vi "FindAltName_wPostfix.vi"(10 "Token":string="__", 11 "File Path Control in":path) -> (3 "File Path Control out":path)   [LabVIEW 2013, in "TestVIs.lvlib"]
doc: "Strips any postfix name from a filename/path. All characters following (and including) the token string are removed. Any file extension is preserved. Token defaults to double-underscore."
uses:
  TestVIs.lvlib
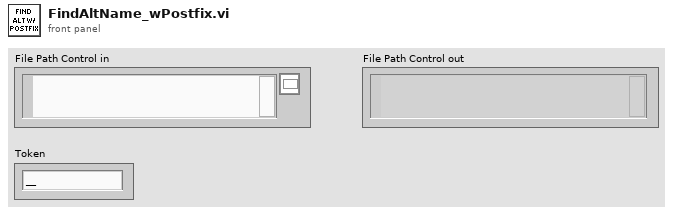
[diagram p1: front panel]
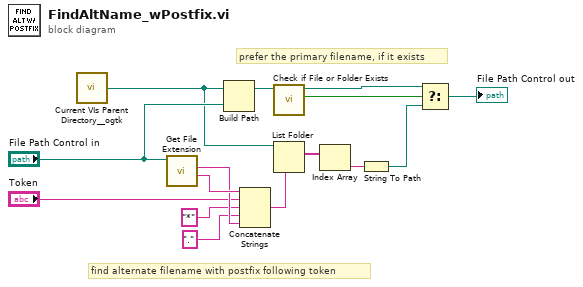
[diagram p0: block diagram]
diagram:
  # "prefer the primary filename, if it exists"
  # "find alternate filename with postfix following token"
  n1 = call <userlib>:"Current VIs Parent Directory__ogtk.vi"() -> ("Parent Directory (+ Relative)"=w5:path)  [unwired: 5 in]
  n2 = call <vilib>:"Get File Extension.vi"("file"="File Path Control in") -> ("filename without extension"=w15:string, "lowercase file extension"=w14:string)  [unwired: 7 in, 2 out]
  n3 = Build Path(base path=w5, name or relative path="File Path Control in") -> (appended path=w7:path)
  n4 = Concatenate Strings(w15, "Token", "*" ("string"), "." ("string"), w14) -> (w12:string)
  n5 = call <vilib>:"Check if File or Folder Exists.vi"("path"=w7) -> ("file or folder exists?"=w4:bool, "dup path"=w3:path)  [unwired: 8 in, 1 out]
  n6 = List Folder(path=w5, pattern=w12) -> (filenames=w11:string[])  [unwired: 2 in, 3 out]
  n7 = Index Array(array=w11) -> (element=w10:string)  [unwired: 1 in]
  n8 = String To Path(string=w10) -> (path=w1:path)
  n9 = Select(t=w3, s=w4, f=w1) -> (s? t:f=→"File Path Control out":path)
